vi "Voorbeeld_Strings.vi"() -> ()   [LabVIEW 2019]
panel:
  out "concatenated string":string
  in  "String 3":string="Deel 2"
  out "length":i32
  out "String 2":string
  in  "String":string="Deel 1"
  in  "stop":bool
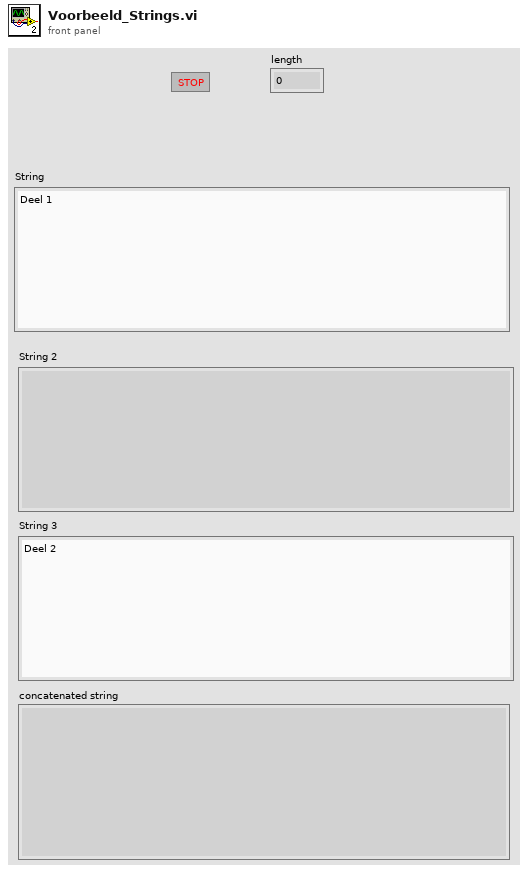
[diagram p1: front panel]
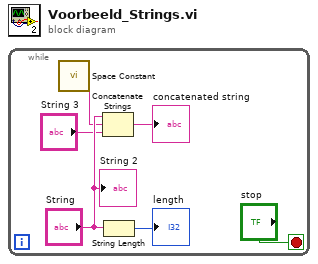
[diagram p0: block diagram]
diagram:
  n1 = while {
    stop <- "stop" stop-if-true
    n2 = call <vilib>:"Space Constant.vi"() -> ("String"=w2:string)
    n3 = Concatenate Strings("String", w2, "String 3") -> (→"concatenated string":string)
    n4 = String Length(string="String") -> (length=→"length":i32)
    "String 2" <- "String"
  }
